vi "Write configuration.vi"(8 "error in":errorcluster, 10 "configuration":refnum<class "NISE_CEF_serializable configuration.lvclass">, 11 "sbRIO-9651 in":refnum<class "sbRIO-9651.lvclass">) -> (0 "error out":errorcluster, 3 "sbRIO-9651 out":refnum<class "sbRIO-9651.lvclass">)   [LabVIEW 2014, in "sbRIO-9651.lvclass"]
uses:
  sbRIO-9651.lvclass
  <vilib>/NI/Configuration Framework/serializable configuration/NISE_CEF_serializable configuration.lvclass
  sbRIO-9651 Configuration.lvclass
  sbRIO-9651.lvclass/sbRIO-9651.ctl
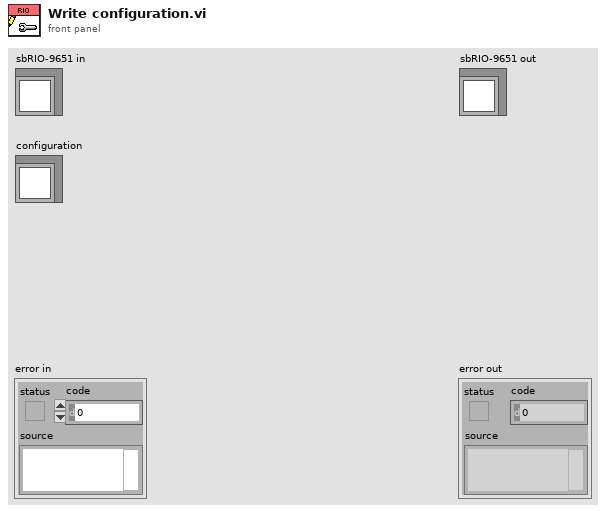
[diagram p1: front panel]
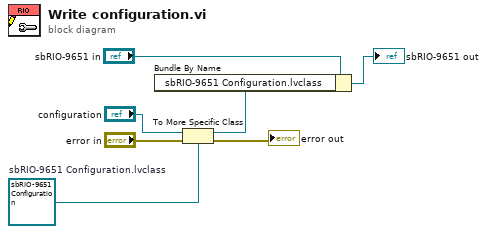
[diagram p0: block diagram]
diagram:
  w1 = refnum<class "sbRIO-9651 Configuration.lvclass"> refnum  # sbRIO-9651 Configuration.lvclass
  n1 = To More Specific Class(target class=w1, reference="configuration", error in="error in") -> (specific class reference=w2:refnum<class "sbRIO-9651 Configuration.lvclass">, error out=→"error out":errorcluster)
  n2 = Bundle By Name(cluster="sbRIO-9651 in", "sbRIO-9651 Configuration.lvclass"=w2) -> (→"sbRIO-9651 out":refnum<class "sbRIO-9651.lvclass">)
